vi "LV Version Number to Year.vi"(10 "VI Version":string) -> (2 "LabVIEW Version":string)   [LabVIEW 2013]
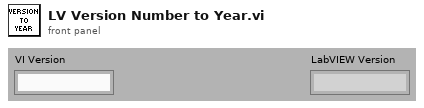
[diagram p1: front panel]
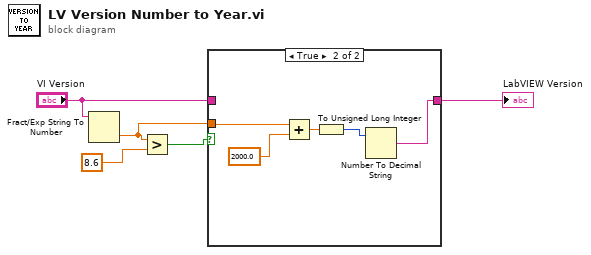
[diagram p0: block diagram]
diagram:
  n1 = Fract/Exp String To Number(string="VI Version") -> (number=w1:dbl)  [unwired: 3 in, 1 out]
  n2 = Greater?(x=w1, y=8.6) -> (0:w4:bool)
  n3 = case shown="True" w4 {
    tunnel: [w6 w7] -> w3
    tunnel: "VI Version" -> [w6 _]
    tunnel: w1 -> [_ w11]
    frame False {
    }
    frame True {
      n4 = Add(x=w11, y=2000.0) -> (x+y=w9:dbl)
      n5 = To Unsigned Long Integer(number=w9) -> (unsigned 32bit integer=w8:u32)
      n6 = Number To Decimal String(number=w8) -> (decimal integer string=w7:string)  [unwired: 1 in]
    }
  }
  "LabVIEW Version" <- w3
